vi "ellipse_zonly_lm_objective.vi"(3 "output control":T1, 4 "data":variant, 5 "X":dbl[](array[numeric]), 6 "a":dbl[](array[numeric])) -> (0 "error out":errorcluster, 1 "f'(X,a)":dbl[][](array[numeric]), 2 "f(X,a)":dbl[](array[numeric]))   [LabVIEW 2017]
doc: "This template is the starting point for creating a model function to be passed to the Nonlinear Curve Fit.vi."
uses:
  <vilib>/gmath/NumericalOptimization/LM_output select.ctl
  typedefs/magnetic field fit.ctl
  <vilib>/gmath/NI_Gmath.lvlib
panel:
  # "a[0] = a, a[1] = b, a[2] = theta, a[3] = B0"
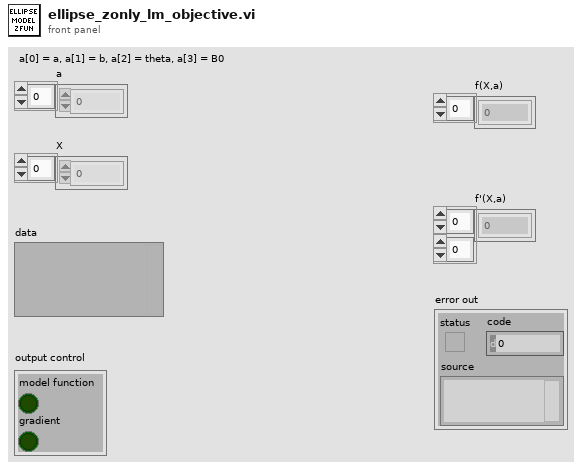
[diagram p1: front panel]
types:
  T1 = typedef "NI_Gmath.lvlib/LM_output select.ctl" = cluster{"model function":bool, "gradient":bool}
  T2 = typedef "magnetic field fit.ctl" = cluster{"a":dbl, "b":dbl, "theta":dbl, "scaling":dbl, "tilt_x":dbl, "tilt_y":dbl, "bx_offset":dbl, "by_offset":dbl, "bz_offset":dbl, "x_offset":dbl, "y_offset":dbl}
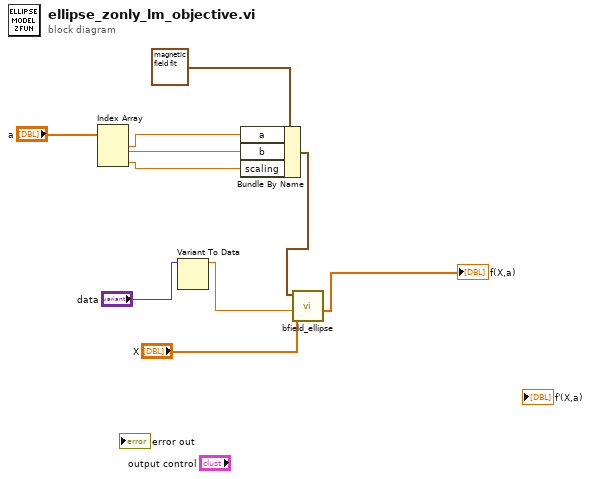
[diagram p0: block diagram]
diagram:
  n1 = Index Array(array="a") -> (element #1=w6:dbl, element #2=w5:dbl, element #3=w4:dbl)  [unwired: 3 in]
  n2 = Variant To Data(Variant="data") -> (data=w9:dbl)  [unwired: 2 in, 1 out]
  n3 = Bundle By Name(cluster=T2 {"a"=0.0, "b"=0.0, "theta"=0.0, "scaling"=0.0, "tilt_x"=0.0, "tilt_y"=0.0, "bx_offset"=0.0, "by_offset"=0.0, "bz_offset"=0.0, "x_offset"=0.0, "y_offset"=0.0} ("parameters"), "a"=w6, "b"=w5, "scaling"=w4) -> (w3:T2)
  n4 = call "bfield_ellipse.vi"("phi"="X", "L"=w9, "parameters"=w3) -> ("Bz"=→"f(X,a)":dbl[])  [unwired: 7 in, 1 out]
